vi "LED_Board_standalone.vi"(0 "LEDs":T1, 1 "Slide":u8(slide)=1 max=31 step=1 scale=0.0..31.0, 2 "White":bool, 3 "Blue":bool, 4 "Green":bool, 5 "Red":bool) -> ()   [LabVIEW 2012]
uses:
  <vilib>/ni845x/ni845x.llb/ni845xControl.ctl
  <vilib>/ni845x/ni845x.llb/NI-845x Close Device Reference.vi
  <resource>/objmgr/NI845x.rc
panel:
  out "Reg0x14":u8 format="%x"
  out "Reg0x13":u8 format="%x"
  out "Reg0x12":u8 format="%x"
  in  "Stop":bool
  out "i2c configuration":refnum<k20>
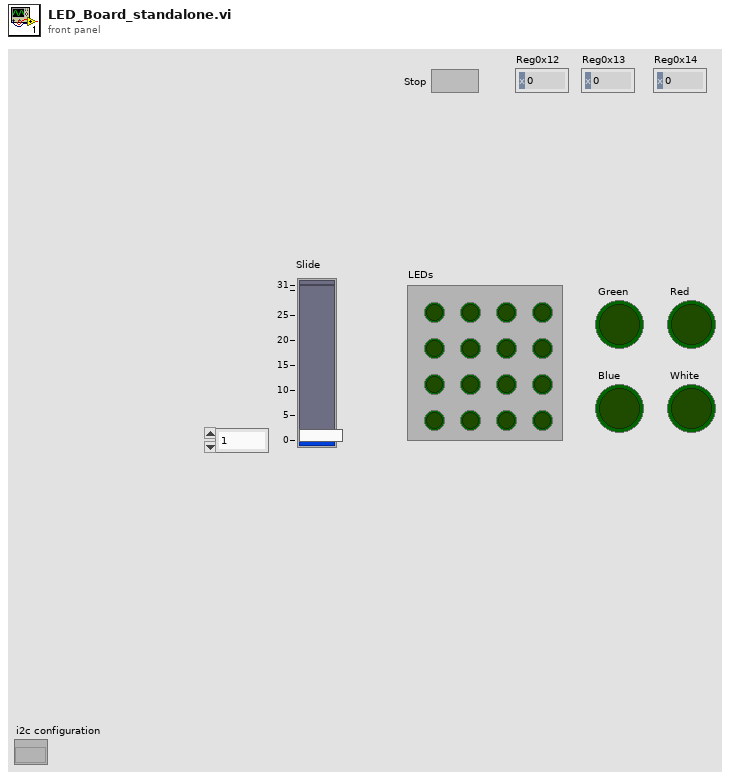
[diagram p1: front panel]
types:
  T1 = cluster{"LED1":bool, "LED2":bool, "LED3":bool, "LED4":bool, "LED5":bool, "LED6":bool, "LED7":bool, "LED8":bool, "LED9":bool, "LED10":bool, "LED11":bool, "LED12":bool, "LED13":bool, "LED14":bool, "LED15":bool, "LED16":bool}
  T2 = typedef "ni845xControl.ctl" = refnum<k21>
  T3 = typedef "ni845xI2cConfiguration.ctl" = refnum<k20>
  T4 = cluster{"[0]":bool, "[1]":bool, "[2]":bool, "[3]":bool, "[4]":bool, "[5]":bool, "[6]":bool, "[7]":bool, "[8]":bool, "[9]":bool, "[10]":bool, "[11]":bool, "[12]":bool, "[13]":bool, "[14]":bool, "[15]":bool}
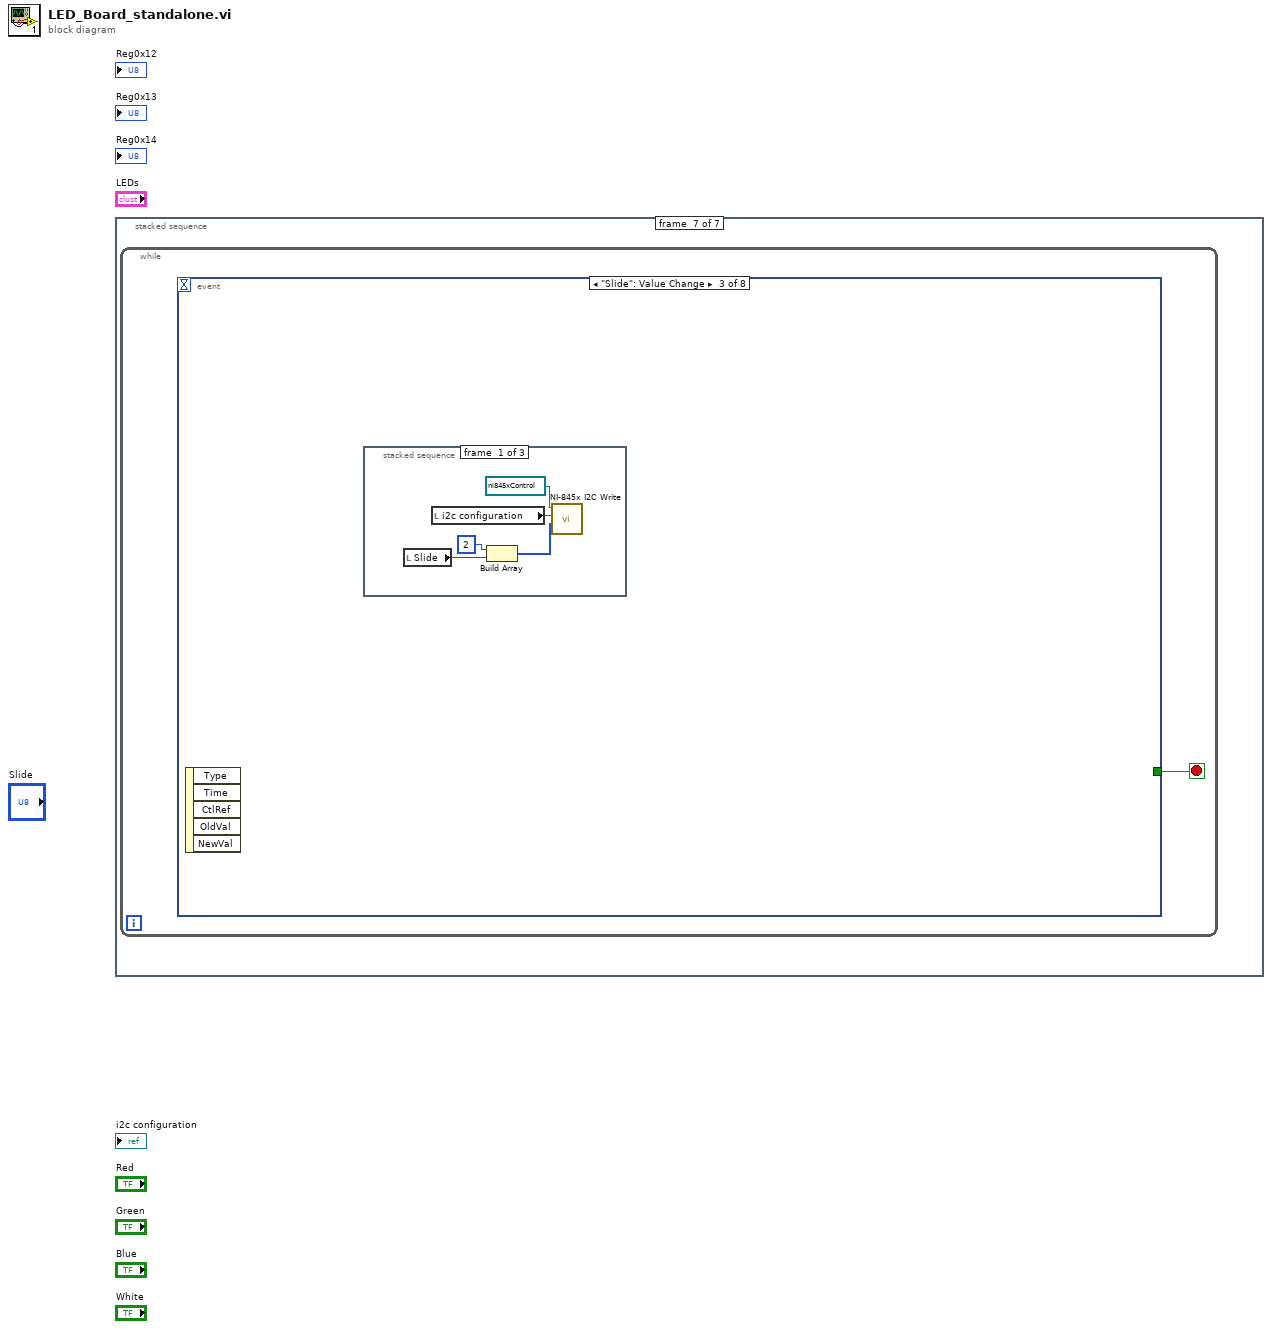
[diagram p0: block diagram]
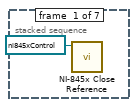
[diagram p2: hidden frame]
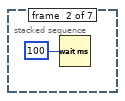
[diagram p3: hidden frame]
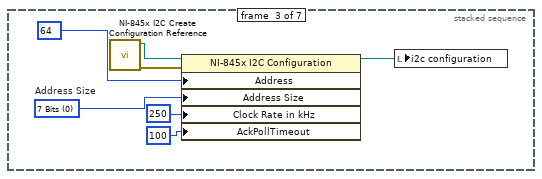
[diagram p4: hidden frame]
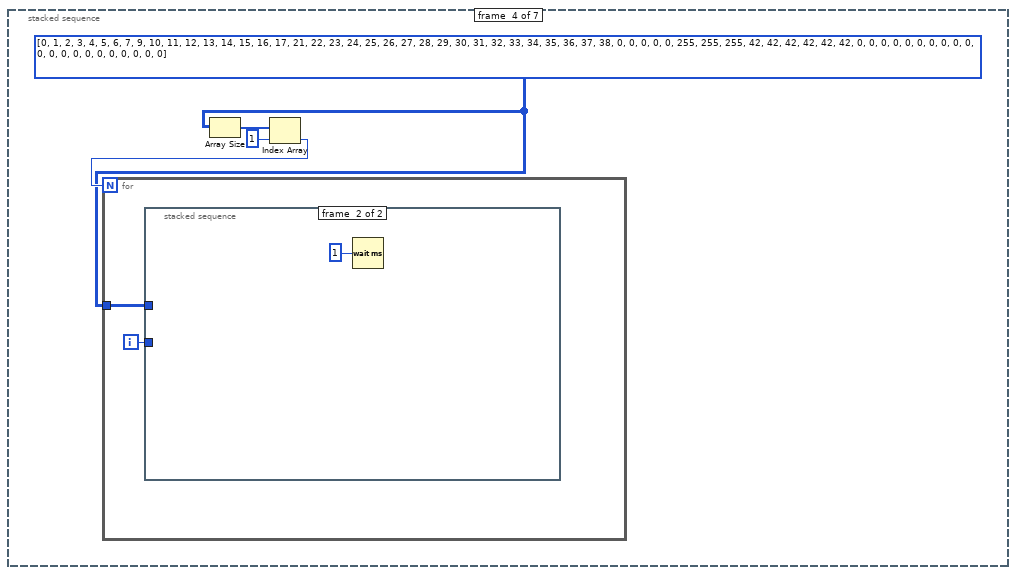
[diagram p5: hidden frame]
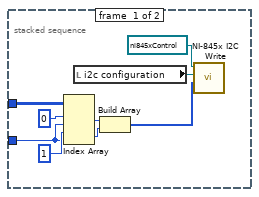
[diagram p6: hidden frame]
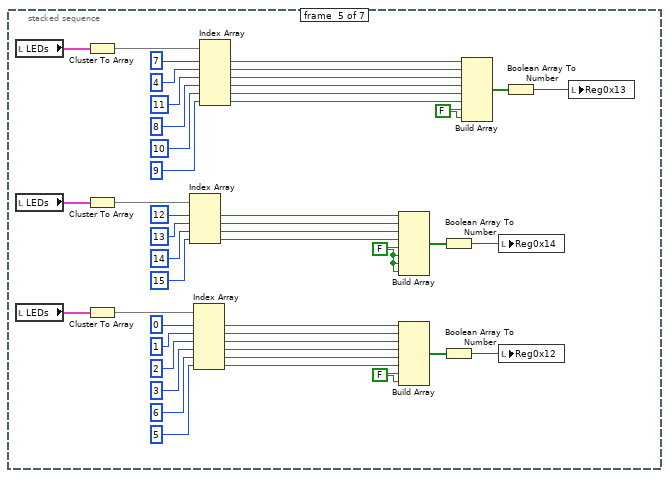
[diagram p7: hidden frame]
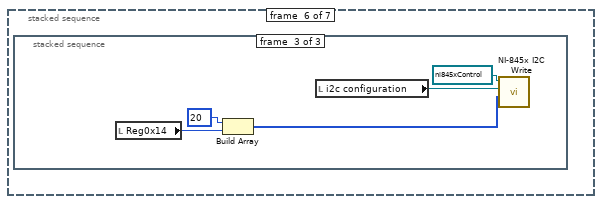
[diagram p8: hidden frame]
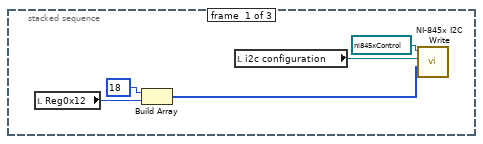
[diagram p9: hidden frame]
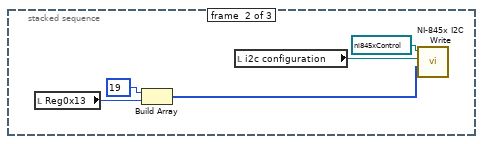
[diagram p10: hidden frame]
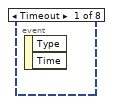
[diagram p11: hidden frame]
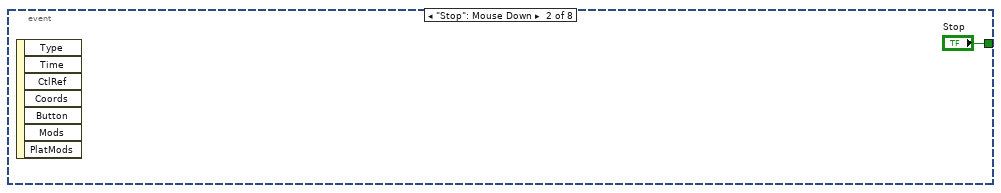
[diagram p12: hidden frame]
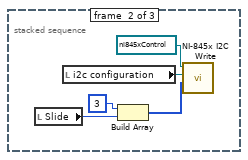
[diagram p13: hidden frame]
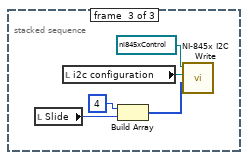
[diagram p14: hidden frame]
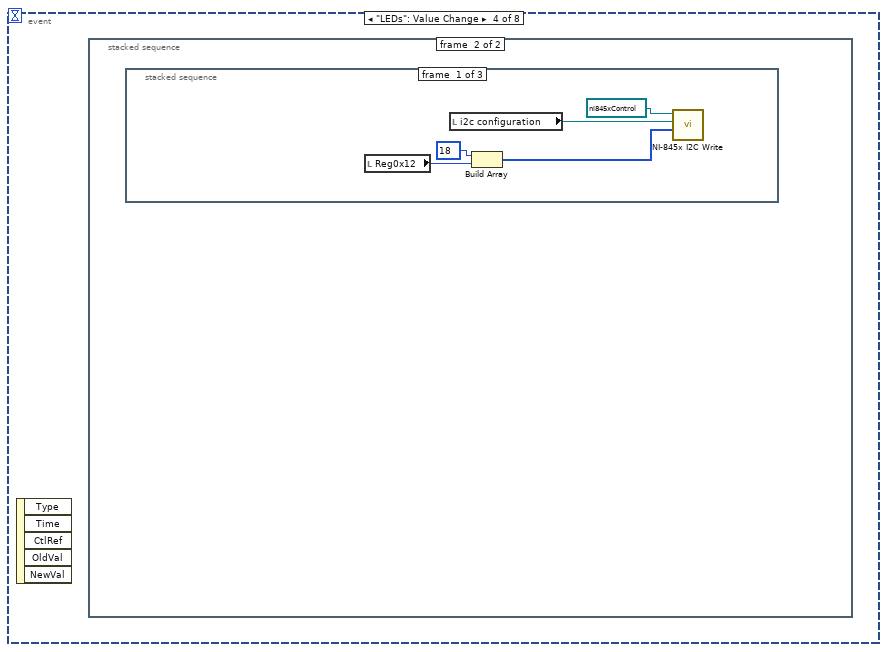
[diagram p15: hidden frame]
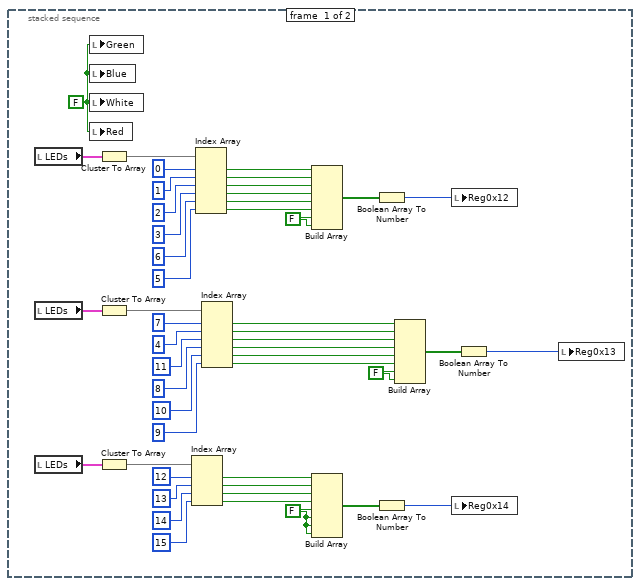
[diagram p16: hidden frame]
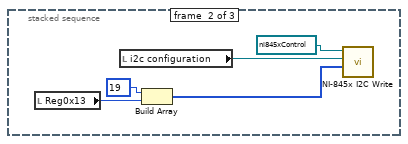
[diagram p17: hidden frame]
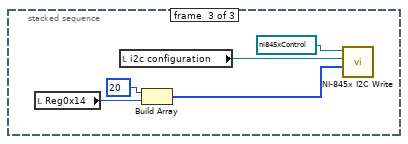
[diagram p18: hidden frame]
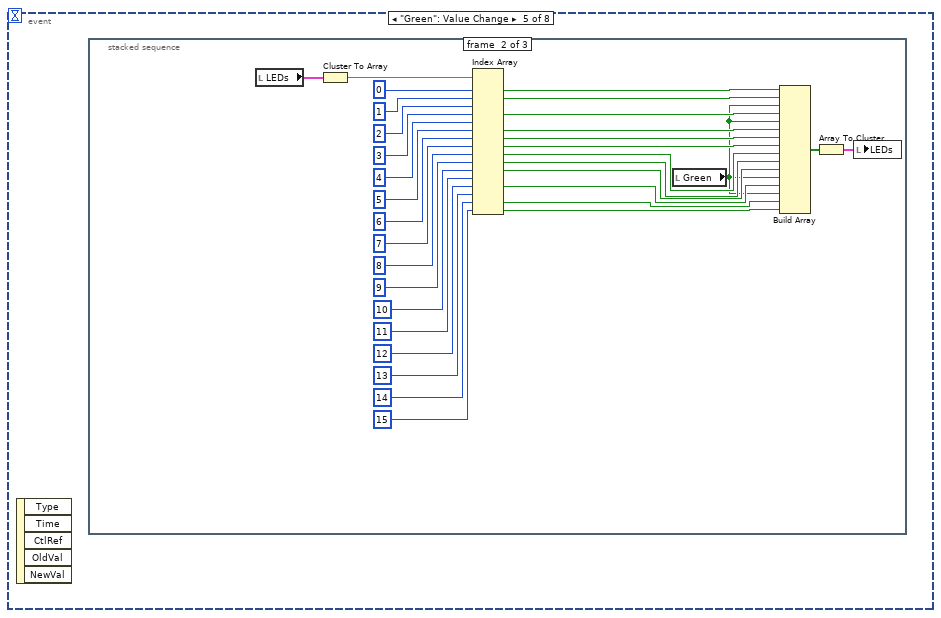
[diagram p19: hidden frame]
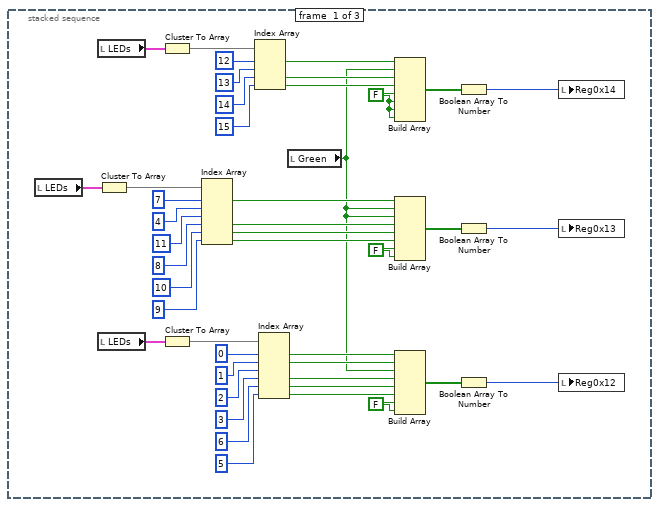
[diagram p20: hidden frame]
diagram:
  n1 = stacked-sequence {
    frame #0 {
      n2 = call-poly <vilib>:"NI-845x Close Reference.vi"("device reference"=T2 "845x") -> ()  [unwired: 10 in, 1 out]
    }
    frame #1 {
      n3 = Wait (ms)(milliseconds to wait=u32 100) -> ()  [unwired: 1 out]
    }
    frame #2 {
      w7 = 0 items=["7 Bits", "10 Bits"]  # Address Size
      n4 = call <vilib>:"NI-845x I2C Create Configuration Reference.vi"() -> ("error out"=w5:errorcluster, "i2c configuration"=w4:T3)  [unwired: 10 in]
      n5 = property on="Property Node" class="NI-845x I2C Configuration"(reference=w4, error in=w5, "Address"=u16 64 ("I2C Address"), "Address Size"=w7, "Clock Rate in kHz"=u16 250, "AckPollTimeout"=u16 100 ("ACK Poll Timeout")) -> (reference out=w8:T3)  [unwired: 1 out]
      n6 = local write "i2c configuration"(w8) -> ()
    }
    frame #3 {
      w10 = u8[][] [[0, 1, 2, 3, 4, 5, 6, 7, 9, 10, 11, 12, 13, 14, 15, 16, 17, 21, 22, 23, 24, 25, 26, 27, 28, 29, 30, 31, 32, 33, 34, 35, 36, 37, 38], [0, 0, 0, 0, 0, 255, 255, 255, 42, 42, 42, 42, 42, 42, 0, 0, 0, 0, 0, 0, 0, 0, 0, 0, 0, 0, 0, 0, 0, 0, 0, 0, 0, 0, 0]] ("Array")
      n7 = Array Size(array=w10) -> (size(s)=w13:i32[])
      n8 = Index Array(array=w13, index=1) -> (element=w11:i32)
      n9 = for {
        N: w11 -> [_]
        tunnel: w10 -> [w15]
        i -> [w14]
        n10 = stacked-sequence {
          tunnel: w15 -> [w24 _]
          tunnel: w14 -> [w21 _]
          frame #0 {
            n11 = Index Array(array=w24, index (row) #1=0 ("index (row)"), index (col) #1=w21, index (row) #2=1 ("index (row)"), index (col) #2=w21) -> (element #1=w18:u8, element #2=w17:u8)
            n12 = local read "i2c configuration"() -> (w19:refnum<k20>)
            n13 = Build Array(w18, w17) -> (w16:u8[])
            n14 = call <vilib>:"NI-845x I2C Write.vi"("write data"=w16, "i2c configuration in"=w19, "device reference in"=T2 "845x" ("device reference")) -> ()  [unwired: 6 in, 3 out]
          }
          frame #1 {
            n15 = Wait (ms)(milliseconds to wait=u32 1) -> ()  [unwired: 1 out]
          }
        }
      }
    }
    frame #4 {
      w29 = FALSE ("element")
      w56 = FALSE ("element")
      w57 = FALSE ("element")
      n16 = local read "LEDs"() -> (w41:T1)
      n17 = local read "LEDs"() -> (w40:T1)
      n18 = local read "LEDs"() -> (w72:T1)
      n19 = Cluster To Array(cluster=w41) -> (array=w44:bool[])
      n20 = Cluster To Array(cluster=w40) -> (array=w37:bool[])
      n21 = Cluster To Array(cluster=w72) -> (array=w69:bool[])
      n22 = Index Array(array=w37, index #1=12 ("index"), index #2=13 ("index"), index #3=14 ("index"), index #4=15 ("index")) -> (element #1=w39:bool, element #2=w33:bool, element #3=w32:bool, element #4=w31:bool)
      n23 = Index Array(array=w69, index #1=0 ("index"), index #2=1 ("index"), index #3=2 ("index"), index #4=3 ("index"), index #5=6 ("index"), index #6=5 ("index")) -> (element #1=w71:bool, element #2=w63:bool, element #3=w62:bool, element #4=w61:bool, element #5=w60:bool, element #6=w59:bool)
      n24 = Index Array(array=w44, index #1=7 ("index"), index #2=4 ("index"), index #3=11 ("index"), index #4=8 ("index"), index #5=10 ("index"), index #6=9 ("index")) -> (element #1=w42:bool, element #2=w50:bool, element #3=w51:bool, element #4=w52:bool, element #5=w53:bool, element #6=w54:bool)
      n25 = Build Array(w39, w33, w32, w31, w29, w29, w29, w29) -> (w30:bool[])
      n26 = Build Array(w71, w63, w62, w61, w60, w59, w57, w57) -> (w58:bool[])
      n27 = Boolean Array To Number(Boolean array=w30) -> (number=w26:u32)
      n28 = Boolean Array To Number(Boolean array=w58) -> (number=w27:u32)
      n29 = Build Array(w42, w50, w51, w52, w53, w54, w56, w56) -> (w55:bool[])
      n30 = local write "Reg0x14"(w26) -> ()
      n31 = local write "Reg0x12"(w27) -> ()
      n32 = Boolean Array To Number(Boolean array=w55) -> (number=w28:u32)
      n33 = local write "Reg0x13"(w28) -> ()
    }
    frame #5 {
      n34 = stacked-sequence {
        frame #0 {
          n35 = local read "Reg0x12"() -> (w75:u8)
          n36 = Build Array(u8 18 ("element"), w75) -> (w73:u8[])
          n37 = local read "i2c configuration"() -> (w77:refnum<k20>)
          n38 = call <vilib>:"NI-845x I2C Write.vi"("write data"=w73, "i2c configuration in"=w77, "device reference in"=T2 "845x" ("device reference")) -> ()  [unwired: 6 in, 3 out]
        }
        frame #1 {
          n39 = local read "Reg0x13"() -> (w80:u8)
          n40 = Build Array(u8 19 ("element"), w80) -> (w78:u8[])
          n41 = local read "i2c configuration"() -> (w82:refnum<k20>)
          n42 = call <vilib>:"NI-845x I2C Write.vi"("write data"=w78, "i2c configuration in"=w82, "device reference in"=T2 "845x" ("device reference")) -> ()  [unwired: 6 in, 3 out]
        }
        frame #2 {
          n43 = local read "Reg0x14"() -> (w85:u8)
          n44 = Build Array(u8 20 ("element"), w85) -> (w83:u8[])
          n45 = local read "i2c configuration"() -> (w87:refnum<k20>)
          n46 = call <vilib>:"NI-845x I2C Write.vi"("write data"=w83, "i2c configuration in"=w87, "device reference in"=T2 "845x" ("device reference")) -> ()  [unwired: 6 in, 3 out]
        }
      }
    }
    frame #6 {
      n47 = while {
        stop <- w88 stop-if-true
        n48 = event shown="[2] \"Slide\": Value Change" {
          selector: _ -> [_ _ _ _ _ _ _ _]
          dyn-events: _ -> [_ _ _ _ _ _ _ _]
          timeout: _ -> [_ _ _ _ _ _ _ _]
          tunnel: [_ "Stop" _ _ _ _ _ _] -> w88
          event Timeout {
            n49 = event-data() -> ()  [unwired: 1 in, 2 out]
          }
          event "Stop": Mouse Down {
            n50 = event-data() -> ()  [unwired: 1 in, 7 out]
          }
          event "Slide": Value Change {
            n51 = event-data() -> ()  [unwired: 1 in, 5 out]
            n52 = stacked-sequence {
              frame #0 {
                n53 = local read "Slide"() -> (w90:u8)
                n54 = local read "i2c configuration"() -> (w94:refnum<k20>)
                n55 = Build Array(u8 2 ("element"), w90) -> (w91:u8[])
                n56 = call <vilib>:"NI-845x I2C Write.vi"("write data"=w91, "i2c configuration in"=w94, "device reference in"=T2 "845x" ("device reference")) -> ()  [unwired: 6 in, 3 out]
              }
              frame #1 {
                n57 = local read "Slide"() -> (w95:u8)
                n58 = local read "i2c configuration"() -> (w99:refnum<k20>)
                n59 = Build Array(u8 3 ("element"), w95) -> (w96:u8[])
                n60 = call <vilib>:"NI-845x I2C Write.vi"("write data"=w96, "i2c configuration in"=w99, "device reference in"=T2 "845x" ("device reference")) -> ()  [unwired: 6 in, 3 out]
              }
              frame #2 {
                n61 = local read "Slide"() -> (w100:u8)
                n62 = local read "i2c configuration"() -> (w104:refnum<k20>)
                n63 = Build Array(u8 4 ("element"), w100) -> (w101:u8[])
                n64 = call <vilib>:"NI-845x I2C Write.vi"("write data"=w101, "i2c configuration in"=w104, "device reference in"=T2 "845x" ("device reference")) -> ()  [unwired: 6 in, 3 out]
              }
            }
          }
          event "LEDs": Value Change {
            n65 = event-data() -> ()  [unwired: 1 in, 5 out]
            n66 = stacked-sequence {
              frame #0 {
                w105 = FALSE ("Green")
                w107 = FALSE ("element")
                w135 = FALSE ("element")
                w137 = FALSE ("element")
                n67 = local read "LEDs"() -> (w152:T1)
                n68 = local read "LEDs"() -> (w120:T1)
                n69 = local read "LEDs"() -> (w118:T1)
                n70 = local write "Green"(w105) -> ()
                n71 = local write "Blue"(w105) -> ()
                n72 = local write "White"(w105) -> ()
                n73 = local write "Red"(w105) -> ()
                n74 = Cluster To Array(cluster=w152) -> (array=w149:bool[])
                n75 = Cluster To Array(cluster=w120) -> (array=w123:bool[])
                n76 = Cluster To Array(cluster=w118) -> (array=w115:bool[])
                n77 = Index Array(array=w115, index #1=12 ("index"), index #2=13 ("index"), index #3=14 ("index"), index #4=15 ("index")) -> (element #1=w117:bool, element #2=w111:bool, element #3=w110:bool, element #4=w109:bool)
                n78 = Index Array(array=w149, index #1=0 ("index"), index #2=1 ("index"), index #3=2 ("index"), index #4=3 ("index"), index #5=6 ("index"), index #6=5 ("index")) -> (element #1=w151:bool, element #2=w143:bool, element #3=w142:bool, element #4=w141:bool, element #5=w140:bool, element #6=w139:bool)
                n79 = Index Array(array=w123, index #1=7 ("index"), index #2=4 ("index"), index #3=11 ("index"), index #4=8 ("index"), index #5=10 ("index"), index #6=9 ("index")) -> (element #1=w121:bool, element #2=w129:bool, element #3=w130:bool, element #4=w131:bool, element #5=w132:bool, element #6=w133:bool)
                n80 = Build Array(w151, w143, w142, w141, w140, w139, w137, w137) -> (w138:bool[])
                n81 = Build Array(w117, w111, w110, w109, w107, w107, w107, w107) -> (w108:bool[])
                n82 = Boolean Array To Number(Boolean array=w138) -> (number=w136:u32)
                n83 = Boolean Array To Number(Boolean array=w108) -> (number=w106:u32)
                n84 = Build Array(w121, w129, w130, w131, w132, w133, w135, w135) -> (w134:bool[])
                n85 = local write "Reg0x12"(w136) -> ()
                n86 = local write "Reg0x14"(w106) -> ()
                n87 = Boolean Array To Number(Boolean array=w134) -> (number=w119:u32)
                n88 = local write "Reg0x13"(w119) -> ()
              }
              frame #1 {
                n89 = stacked-sequence {
                  frame #0 {
                    n90 = local read "Reg0x12"() -> (w155:u8)
                    n91 = local read "i2c configuration"() -> (w157:refnum<k20>)
                    n92 = Build Array(u8 18 ("element"), w155) -> (w153:u8[])
                    n93 = call <vilib>:"NI-845x I2C Write.vi"("write data"=w153, "i2c configuration in"=w157, "device reference in"=T2 "845x" ("device reference")) -> ()  [unwired: 6 in, 3 out]
                  }
                  frame #1 {
                    n94 = local read "Reg0x13"() -> (w160:u8)
                    n95 = local read "i2c configuration"() -> (w162:refnum<k20>)
                    n96 = Build Array(u8 19 ("element"), w160) -> (w158:u8[])
                    n97 = call <vilib>:"NI-845x I2C Write.vi"("write data"=w158, "i2c configuration in"=w162, "device reference in"=T2 "845x" ("device reference")) -> ()  [unwired: 6 in, 3 out]
                  }
                  frame #2 {
                    n98 = local read "Reg0x14"() -> (w165:u8)
                    n99 = local read "i2c configuration"() -> (w167:refnum<k20>)
                    n100 = Build Array(u8 20 ("element"), w165) -> (w163:u8[])
                    n101 = call <vilib>:"NI-845x I2C Write.vi"("write data"=w163, "i2c configuration in"=w167, "device reference in"=T2 "845x" ("device reference")) -> ()  [unwired: 6 in, 3 out]
                  }
                }
              }
            }
          }
          event "Green": Value Change {
            n102 = event-data() -> ()  [unwired: 1 in, 5 out]
            n103 = stacked-sequence {
              frame #0 {
                w172 = FALSE ("element")
                w196 = FALSE ("element")
                w198 = FALSE ("element")
                n104 = local read "LEDs"() -> (w183:T1)
                n105 = local read "LEDs"() -> (w181:T1)
                n106 = local read "LEDs"() -> (w211:T1)
                n107 = Cluster To Array(cluster=w183) -> (array=w186:bool[])
                n108 = Cluster To Array(cluster=w181) -> (array=w178:bool[])
                n109 = Cluster To Array(cluster=w211) -> (array=w208:bool[])
                n110 = Index Array(array=w186, index #1=7 ("index"), index #2=4 ("index"), index #3=11 ("index"), index #4=8 ("index"), index #5=10 ("index"), index #6=9 ("index")) -> (element #1=w184:bool, element #4=w192:bool, element #5=w193:bool, element #6=w194:bool)  [unwired: 2 out]
                n111 = Index Array(array=w178, index #1=12 ("index"), index #2=13 ("index"), index #3=14 ("index"), index #4=15 ("index")) -> (element #1=w180:bool, element #3=w169:bool, element #4=w174:bool)  [unwired: 1 out]
                n112 = Index Array(array=w208, index #1=0 ("index"), index #2=1 ("index"), index #3=2 ("index"), index #4=3 ("index"), index #5=6 ("index"), index #6=5 ("index")) -> (element #1=w210:bool, element #2=w170:bool, element #4=w202:bool, element #5=w201:bool, element #6=w200:bool)  [unwired: 1 out]
                n113 = local read "Green"() -> (w168:bool)
                n114 = Build Array(w180, w168, w169, w174, w172, w172, w172, w172) -> (w173:bool[])
                n115 = Build Array(w184, w168, w168, w192, w193, w194, w196, w196) -> (w195:bool[])
                n116 = Build Array(w210, w170, w168, w202, w201, w200, w198, w198) -> (w199:bool[])
                n117 = Boolean Array To Number(Boolean array=w173) -> (number=w171:u32)
                n118 = Boolean Array To Number(Boolean array=w195) -> (number=w182:u32)
                n119 = Boolean Array To Number(Boolean array=w199) -> (number=w197:u32)
                n120 = local write "Reg0x14"(w171) -> ()
                n121 = local write "Reg0x13"(w182) -> ()
                n122 = local write "Reg0x12"(w197) -> ()
              }
              frame #1 {
                n123 = local read "LEDs"() -> (w244:T1)
                n124 = Cluster To Array(cluster=w244) -> (array=w243:bool[])
                n125 = Index Array(array=w243, index #1=0 ("index"), index #2=1 ("index"), index #3=2 ("index"), index #4=3 ("index"), index #5=4 ("index"), index #6=5 ("index"), index #7=6 ("index"), index #8=7 ("index"), index #9=8 ("index"), index #10=9 ("index"), index #11=10 ("index"), index #12=11 ("index"), index #13=12 ("index"), index #14=13 ("index"), index #15=14 ("index"), index #16=15 ("index")) -> (element #1=w215:bool, element #2=w216:bool, element #4=w217:bool, element #6=w218:bool, element #7=w219:bool, element #8=w220:bool, element #9=w221:bool, element #10=w222:bool, element #11=w223:bool, element #13=w224:bool, element #15=w225:bool, element #16=w226:bool)  [unwired: 4 out]
                n126 = local read "Green"() -> (w214:bool)
                n127 = Build Array(w215, w216, w214, w217, w214, w218, w219, w220, w221, w222, w223, w214, w224, w214, w225, w226) -> (w213:bool[])
                n128 = Array To Cluster(array=w213) -> (cluster=w212:T4)
                n129 = local write "LEDs"(w212) -> ()
              }
              frame #2 {
                n130 = stacked-sequence {
                  frame #0 {
                    n131 = local read "Reg0x12"() -> (w247:u8)
                    n132 = local read "i2c configuration"() -> (w249:refnum<k20>)
                    n133 = Build Array(u8 18 ("element"), w247) -> (w245:u8[])
                    n134 = call <vilib>:"NI-845x I2C Write.vi"("write data"=w245, "i2c configuration in"=w249, "device reference in"=T2 "845x" ("device reference")) -> ()  [unwired: 6 in, 3 out]
                  }
                  frame #1 {
                    n135 = local read "Reg0x13"() -> (w252:u8)
                    n136 = local read "i2c configuration"() -> (w254:refnum<k20>)
                    n137 = Build Array(u8 19 ("element"), w252) -> (w250:u8[])
                    n138 = call <vilib>:"NI-845x I2C Write.vi"("write data"=w250, "i2c configuration in"=w254, "device reference in"=T2 "845x" ("device reference")) -> ()  [unwired: 6 in, 3 out]
                  }
                  frame #2 {
                    n139 = local read "Reg0x14"() -> (w257:u8)
                    n140 = local read "i2c configuration"() -> (w259:refnum<k20>)
                    n141 = Build Array(u8 20 ("element"), w257) -> (w255:u8[])
                    n142 = call <vilib>:"NI-845x I2C Write.vi"("write data"=w255, "i2c configuration in"=w259, "device reference in"=T2 "845x" ("device reference")) -> ()  [unwired: 6 in, 3 out]
                  }
                }
              }
            }
          }
          event "Red": Value Change {
            n143 = event-data() -> ()  [unwired: 1 in, 5 out]
            n144 = stacked-sequence {
              frame #0 {
                w265 = FALSE ("element")
                w288 = FALSE ("element")
                w290 = FALSE ("element")
                n145 = local read "LEDs"() -> (w277:T1)
                n146 = local read "LEDs"() -> (w275:T1)
                n147 = local read "LEDs"() -> (w303:T1)
                n148 = Cluster To Array(cluster=w277) -> (array=w279:bool[])
                n149 = Cluster To Array(cluster=w275) -> (array=w272:bool[])
                n150 = Cluster To Array(cluster=w303) -> (array=w300:bool[])
                n151 = Index Array(array=w279, index #1=7 ("index"), index #2=4 ("index"), index #3=11 ("index"), index #4=8 ("index"), index #5=10 ("index"), index #6=9 ("index")) -> (element #2=w261:bool, element #3=w262:bool, element #5=w285:bool, element #6=w286:bool)  [unwired: 2 out]
                n152 = Index Array(array=w272, index #1=12 ("index"), index #2=13 ("index"), index #3=14 ("index"), index #4=15 ("index")) -> (element #1=w274:bool, element #2=w268:bool, element #4=w267:bool)  [unwired: 1 out]
                n153 = Index Array(array=w300, index #1=0 ("index"), index #2=1 ("index"), index #3=2 ("index"), index #4=3 ("index"), index #5=6 ("index"), index #6=5 ("index")) -> (element #1=w302:bool, element #3=w263:bool, element #4=w294:bool, element #5=w293:bool, element #6=w292:bool)  [unwired: 1 out]
                n154 = local read "Red"() -> (w260:bool)
                n155 = Build Array(w274, w268, w260, w267, w265, w265, w265, w265) -> (w266:bool[])
                n156 = Build Array(w260, w261, w262, w260, w285, w286, w288, w288) -> (w287:bool[])
                n157 = Build Array(w302, w260, w263, w294, w293, w292, w290, w290) -> (w291:bool[])
                n158 = Boolean Array To Number(Boolean array=w266) -> (number=w264:u32)
                n159 = Boolean Array To Number(Boolean array=w287) -> (number=w276:u32)
                n160 = Boolean Array To Number(Boolean array=w291) -> (number=w289:u32)
                n161 = local write "Reg0x14"(w264) -> ()
                n162 = local write "Reg0x13"(w276) -> ()
                n163 = local write "Reg0x12"(w289) -> ()
              }
              frame #1 {
                n164 = local read "LEDs"() -> (w336:T1)
                n165 = Cluster To Array(cluster=w336) -> (array=w335:bool[])
                n166 = Index Array(array=w335, index #1=0 ("index"), index #2=1 ("index"), index #3=2 ("index"), index #4=3 ("index"), index #5=4 ("index"), index #6=5 ("index"), index #7=6 ("index"), index #8=7 ("index"), index #9=8 ("index"), index #10=9 ("index"), index #11=10 ("index"), index #12=11 ("index"), index #13=12 ("index"), index #14=13 ("index"), index #15=14 ("index"), index #16=15 ("index")) -> (element #1=w311:bool, element #3=w308:bool, element #4=w312:bool, element #5=w307:bool, element #6=w313:bool, element #7=w314:bool, element #10=w315:bool, element #11=w316:bool, element #12=w306:bool, element #13=w317:bool, element #14=w305:bool, element #16=w318:bool)  [unwired: 4 out]
                n167 = local read "Red"() -> (w304:bool)
                n168 = Build Array(w311, w304, w308, w312, w307, w313, w314, w304, w304, w315, w316, w306, w317, w305, w304, w318) -> (w310:bool[])
                n169 = Array To Cluster(array=w310) -> (cluster=w309:T4)
                n170 = local write "LEDs"(w309) -> ()
              }
              frame #2 {
                n171 = stacked-sequence {
                  frame #0 {
                    n172 = local read "Reg0x12"() -> (w339:u8)
                    n173 = local read "i2c configuration"() -> (w341:refnum<k20>)
                    n174 = Build Array(u8 18 ("element"), w339) -> (w337:u8[])
                    n175 = call <vilib>:"NI-845x I2C Write.vi"("write data"=w337, "i2c configuration in"=w341, "device reference in"=T2 "845x" ("device reference")) -> ()  [unwired: 6 in, 3 out]
                  }
                  frame #1 {
                    n176 = local read "Reg0x13"() -> (w344:u8)
                    n177 = local read "i2c configuration"() -> (w346:refnum<k20>)
                    n178 = Build Array(u8 19 ("element"), w344) -> (w342:u8[])
                    n179 = call <vilib>:"NI-845x I2C Write.vi"("write data"=w342, "i2c configuration in"=w346, "device reference in"=T2 "845x" ("device reference")) -> ()  [unwired: 6 in, 3 out]
                  }
                  frame #2 {
                    n180 = local read "Reg0x14"() -> (w349:u8)
                    n181 = local read "i2c configuration"() -> (w351:refnum<k20>)
                    n182 = Build Array(u8 20 ("element"), w349) -> (w347:u8[])
                    n183 = call <vilib>:"NI-845x I2C Write.vi"("write data"=w347, "i2c configuration in"=w351, "device reference in"=T2 "845x" ("device reference")) -> ()  [unwired: 6 in, 3 out]
                  }
                }
              }
            }
          }
          event "Blue": Value Change {
            n184 = event-data() -> ()  [unwired: 1 in, 5 out]
            n185 = stacked-sequence {
              frame #0 {
                w361 = FALSE ("element")
                w382 = FALSE ("element")
                w384 = FALSE ("element")
                n186 = local read "LEDs"() -> (w371:T1)
                n187 = local read "LEDs"() -> (w373:T1)
                n188 = local read "LEDs"() -> (w395:T1)
                n189 = Cluster To Array(cluster=w371) -> (array=w368:bool[])
                n190 = Cluster To Array(cluster=w373) -> (array=w375:bool[])
                n191 = Cluster To Array(cluster=w395) -> (array=w392:bool[])
                n192 = Index Array(array=w368, index #1=12 ("index"), index #2=13 ("index"), index #3=14 ("index"), index #4=15 ("index")) -> (element #1=w370:bool, element #2=w364:bool, element #3=w353:bool, element #4=w363:bool)
                n193 = Index Array(array=w375, index #1=7 ("index"), index #2=4 ("index"), index #3=11 ("index"), index #4=8 ("index"), index #5=10 ("index"), index #6=9 ("index")) -> (element #1=w355:bool, element #2=w357:bool, element #3=w358:bool, element #4=w354:bool)  [unwired: 2 out]
                n194 = Index Array(array=w392, index #1=0 ("index"), index #2=1 ("index"), index #3=2 ("index"), index #4=3 ("index"), index #5=6 ("index"), index #6=5 ("index")) -> (element #1=w394:bool, element #2=w356:bool, element #3=w359:bool, element #4=w386:bool)  [unwired: 2 out]
                n195 = local read "Blue"() -> (w352:bool)
                n196 = Build Array(w370, w364, w353, w363, w361, w361, w361, w361) -> (w362:bool[])
                n197 = Boolean Array To Number(Boolean array=w362) -> (number=w360:u32)
                n198 = Build Array(w355, w357, w358, w354, w352, w352, w382, w382) -> (w381:bool[])
                n199 = Build Array(w394, w356, w359, w386, w352, w352, w384, w384) -> (w385:bool[])
                n200 = local write "Reg0x14"(w360) -> ()
                n201 = Boolean Array To Number(Boolean array=w381) -> (number=w372:u32)
                n202 = Boolean Array To Number(Boolean array=w385) -> (number=w383:u32)
                n203 = local write "Reg0x13"(w372) -> ()
                n204 = local write "Reg0x12"(w383) -> ()
              }
              frame #1 {
                n205 = local read "LEDs"() -> (w428:T1)
                n206 = Cluster To Array(cluster=w428) -> (array=w427:bool[])
                n207 = Index Array(array=w427, index #1=0 ("index"), index #2=1 ("index"), index #3=2 ("index"), index #4=3 ("index"), index #5=4 ("index"), index #6=5 ("index"), index #7=6 ("index"), index #8=7 ("index"), index #9=8 ("index"), index #10=9 ("index"), index #11=10 ("index"), index #12=11 ("index"), index #13=12 ("index"), index #14=13 ("index"), index #15=14 ("index"), index #16=15 ("index")) -> (element #1=w403:bool, element #2=w404:bool, element #3=w400:bool, element #4=w405:bool, element #5=w399:bool, element #8=w406:bool, element #9=w407:bool, element #12=w398:bool, element #13=w408:bool, element #14=w397:bool, element #15=w409:bool, element #16=w410:bool)  [unwired: 4 out]
                n208 = local read "Blue"() -> (w396:bool)
                n209 = Build Array(w403, w404, w400, w405, w399, w396, w396, w406, w407, w396, w396, w398, w408, w397, w409, w410) -> (w402:bool[])
                n210 = Array To Cluster(array=w402) -> (cluster=w401:T4)
                n211 = local write "LEDs"(w401) -> ()
              }
              frame #2 {
                n212 = stacked-sequence {
                  frame #0 {
                    n213 = local read "Reg0x12"() -> (w431:u8)
                    n214 = local read "i2c configuration"() -> (w433:refnum<k20>)
                    n215 = Build Array(u8 18 ("element"), w431) -> (w429:u8[])
                    n216 = call <vilib>:"NI-845x I2C Write.vi"("write data"=w429, "i2c configuration in"=w433, "device reference in"=T2 "845x" ("device reference")) -> ()  [unwired: 6 in, 3 out]
                  }
                  frame #1 {
                    n217 = local read "Reg0x13"() -> (w436:u8)
                    n218 = local read "i2c configuration"() -> (w438:refnum<k20>)
                    n219 = Build Array(u8 19 ("element"), w436) -> (w434:u8[])
                    n220 = call <vilib>:"NI-845x I2C Write.vi"("write data"=w434, "i2c configuration in"=w438, "device reference in"=T2 "845x" ("device reference")) -> ()  [unwired: 6 in, 3 out]
                  }
                  frame #2 {
                    n221 = local read "Reg0x14"() -> (w441:u8)
                    n222 = local read "i2c configuration"() -> (w443:refnum<k20>)
                    n223 = Build Array(u8 20 ("element"), w441) -> (w439:u8[])
                    n224 = call <vilib>:"NI-845x I2C Write.vi"("write data"=w439, "i2c configuration in"=w443, "device reference in"=T2 "845x" ("device reference")) -> ()  [unwired: 6 in, 3 out]
                  }
                }
              }
            }
          }
          event "White": Value Change {
            n225 = event-data() -> ()  [unwired: 1 in, 5 out]
            n226 = stacked-sequence {
              frame #0 {
                w457 = FALSE ("element")
                w476 = FALSE ("element")
                w478 = FALSE ("element")
                n227 = local read "LEDs"() -> (w465:T1)
                n228 = local read "LEDs"() -> (w487:T1)
                n229 = local read "LEDs"() -> (w467:T1)
                n230 = Cluster To Array(cluster=w465) -> (array=w463:bool[])
                n231 = Cluster To Array(cluster=w487) -> (array=w485:bool[])
                n232 = Cluster To Array(cluster=w467) -> (array=w469:bool[])
                n233 = Index Array(array=w463, index #1=12 ("index"), index #2=13 ("index"), index #3=14 ("index"), index #4=15 ("index")) -> (element #2=w459:bool, element #3=w449:bool)  [unwired: 2 out]
                n234 = Index Array(array=w485, index #1=0 ("index"), index #2=1 ("index"), index #3=2 ("index"), index #4=3 ("index"), index #5=6 ("index"), index #6=5 ("index")) -> (element #2=w452:bool, element #3=w455:bool, element #5=w446:bool, element #6=w445:bool)  [unwired: 2 out]
                n235 = Index Array(array=w469, index #1=7 ("index"), index #2=4 ("index"), index #3=11 ("index"), index #4=8 ("index"), index #5=10 ("index"), index #6=9 ("index")) -> (element #1=w451:bool, element #2=w453:bool, element #3=w454:bool, element #4=w450:bool, element #5=w448:bool, element #6=w447:bool)
                n236 = local read "White"() -> (w444:bool)
                n237 = Build Array(w444, w459, w449, w444, w457, w457, w457, w457) -> (w458:bool[])
                n238 = Build Array(w444, w452, w455, w444, w446, w445, w478, w478) -> (w479:bool[])
                n239 = Boolean Array To Number(Boolean array=w458) -> (number=w456:u32)
                n240 = Boolean Array To Number(Boolean array=w479) -> (number=w477:u32)
                n241 = Build Array(w451, w453, w454, w450, w448, w447, w476, w476) -> (w475:bool[])
                n242 = local write "Reg0x14"(w456) -> ()
                n243 = local write "Reg0x12"(w477) -> ()
                n244 = Boolean Array To Number(Boolean array=w475) -> (number=w466:u32)
                n245 = local write "Reg0x13"(w466) -> ()
              }
              frame #1 {
                n246 = local read "LEDs"() -> (w520:T1)
                n247 = Cluster To Array(cluster=w520) -> (array=w519:bool[])
                n248 = Index Array(array=w519, index #1=0 ("index"), index #2=1 ("index"), index #3=2 ("index"), index #4=3 ("index"), index #5=4 ("index"), index #6=5 ("index"), index #7=6 ("index"), index #8=7 ("index"), index #9=8 ("index"), index #10=9 ("index"), index #11=10 ("index"), index #12=11 ("index"), index #13=12 ("index"), index #14=13 ("index"), index #15=14 ("index"), index #16=15 ("index")) -> (element #2=w499:bool, element #3=w496:bool, element #5=w495:bool, element #6=w492:bool, element #7=w491:bool, element #8=w500:bool, element #9=w501:bool, element #10=w490:bool, element #11=w489:bool, element #12=w494:bool, element #14=w493:bool, element #15=w502:bool)  [unwired: 4 out]
                n249 = local read "White"() -> (w488:bool)
                n250 = Build Array(w488, w499, w496, w488, w495, w492, w491, w500, w501, w490, w489, w494, w488, w493, w502, w488) -> (w498:bool[])
                n251 = Array To Cluster(array=w498) -> (cluster=w497:T4)
                n252 = local write "LEDs"(w497) -> ()
              }
              frame #2 {
                n253 = stacked-sequence {
                  frame #0 {
                    n254 = local read "Reg0x12"() -> (w523:u8)
                    n255 = local read "i2c configuration"() -> (w525:refnum<k20>)
                    n256 = Build Array(u8 18 ("element"), w523) -> (w521:u8[])
                    n257 = call <vilib>:"NI-845x I2C Write.vi"("write data"=w521, "i2c configuration in"=w525, "device reference in"=T2 "845x" ("device reference")) -> ()  [unwired: 6 in, 3 out]
                  }
                  frame #1 {
                    n258 = local read "Reg0x13"() -> (w528:u8)
                    n259 = local read "i2c configuration"() -> (w530:refnum<k20>)
                    n260 = Build Array(u8 19 ("element"), w528) -> (w526:u8[])
                    n261 = call <vilib>:"NI-845x I2C Write.vi"("write data"=w526, "i2c configuration in"=w530, "device reference in"=T2 "845x" ("device reference")) -> ()  [unwired: 6 in, 3 out]
                  }
                  frame #2 {
                    n262 = local read "Reg0x14"() -> (w533:u8)
                    n263 = local read "i2c configuration"() -> (w535:refnum<k20>)
                    n264 = Build Array(u8 20 ("element"), w533) -> (w531:u8[])
                    n265 = call <vilib>:"NI-845x I2C Write.vi"("write data"=w531, "i2c configuration in"=w535, "device reference in"=T2 "845x" ("device reference")) -> ()  [unwired: 6 in, 3 out]
                  }
                }
              }
            }
          }
        }
      }
    }
  }
